vi "Robot Move Board.vi"(9 "Z":dbl, 10 "Value":T1, 11 "Laser Point":cluster{"X":dbl, "Y":dbl, "Angle":dbl}) -> (0 "error out":errorcluster)   [LabVIEW 2019, in "MPC_Laser Marked.lvclass"]
uses:
  MPC_Laser Marked.lvclass
  Function/Main UI/Ctrl/XY Table Action.ctl
  LLB/Commonly VI/FilterPointNameToFloat.vi
  Function/Axis/Axis_Class/SubVI/Axis Motion/Axis_Go Point.vi
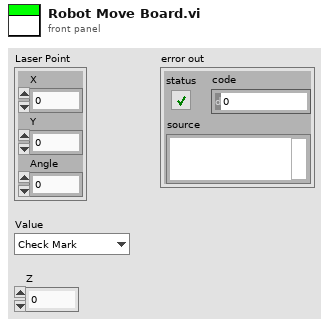
[diagram p1: front panel]
types:
  T1 = typedef "XY Table Action.ctl" = enum16{"Check Mark", "Check Z", "Laser", "Request Action"}
  T2 = enum16{"Initial", "Load", "Save", "Read", "WriteSpeed", "WritePoint"}
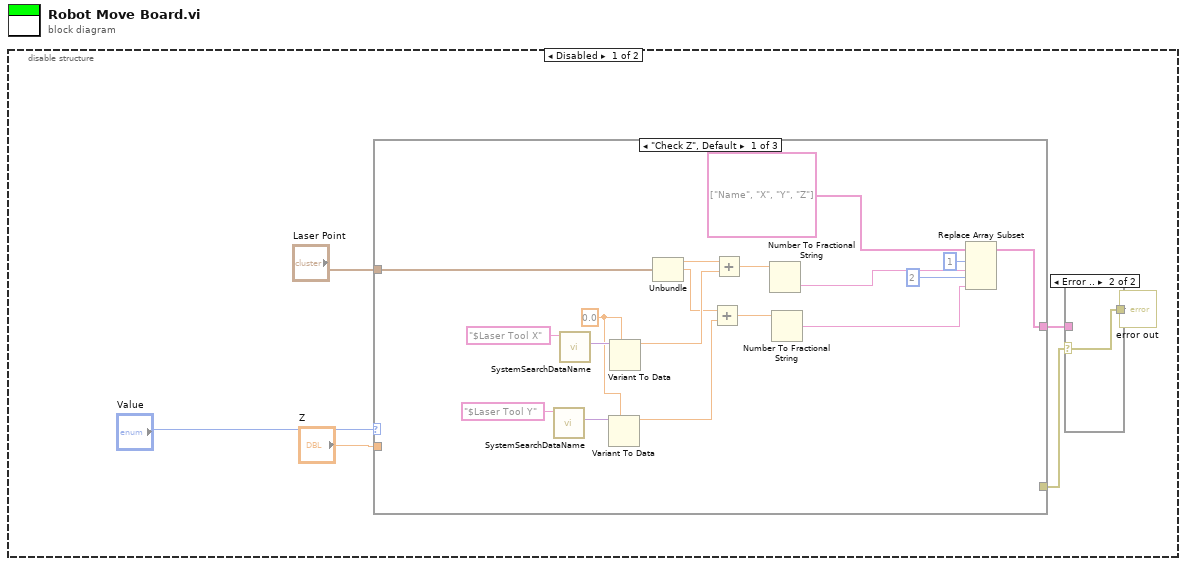
[diagram p0: block diagram]
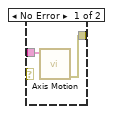
[diagram p2: hidden frame]
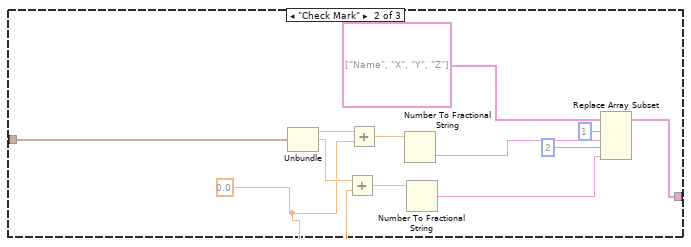
[diagram p3: hidden frame]
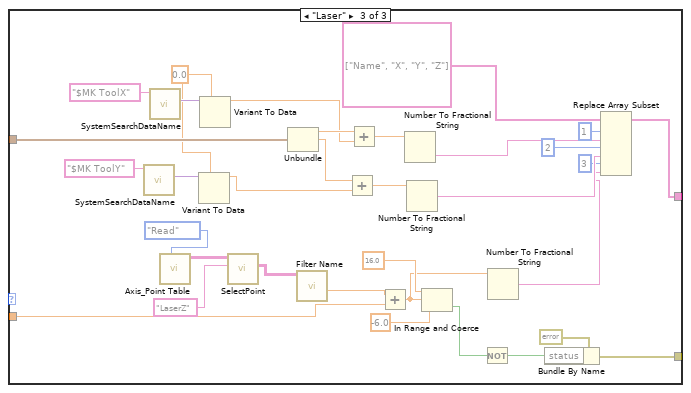
[diagram p4: hidden frame]
diagram:
  n1 = disable-structure shown="Disabled" {
    frame Disabled {
      n2 = case shown="\"Check Z\", Default" "Value" {
        tunnel: [w17 w36 w69] -> w1
        tunnel: "Laser Point" -> [w10 w29 w62]
        tunnel: "Z" -> [_ _ w56]
        tunnel: [_ _ w52] -> w6
        frame "Check Z", Default {
          w23 = 0.0
          n3 = call "SystemSearchDataName.vi"("element"="$Laser Tool Y") -> ("variant"=w24:variant)  [unwired: 8 in, 2 out]
          n4 = call "SystemSearchDataName.vi"("element"="$Laser Tool X") -> ("variant"=w25:variant)  [unwired: 8 in, 2 out]
          n5 = Variant To Data(type=w23, Variant=w24) -> (data=w19:dbl)  [unwired: 1 in, 1 out]
          n6 = Variant To Data(type=w23, Variant=w25) -> (data=w21:dbl)  [unwired: 1 in, 1 out]
          n7 = Unbundle(w10) -> ("X"=w22:dbl, "Y"=w20:dbl)  [unwired: 1 out]
          n8 = Add(x=w20, y=w19) -> (x+y=w15:dbl)
          n9 = Add(x=w22, y=w21) -> (x+y=w16:dbl)
          n10 = Number To Fractional String(number=w16) -> (F-format string=w12:string)  [unwired: 3 in]
          n11 = Number To Fractional String(number=w15) -> (F-format string=w11:string)  [unwired: 3 in]
          n12 = Replace Array Subset(array=string[] ["Name", "X", "Y", "Z"] ("RobotPointsOut"), new element #1=w12, index #1=1 ("index"), new element #2=w11, index #2=2 ("index")) -> (w17:string[])
        }
        frame "Check Mark" {
          w28 = 0.0
          n13 = Unbundle(w29) -> ("X"=w39:dbl, "Y"=w38:dbl)  [unwired: 1 out]
          n14 = Add(x=w38, y=w28) -> (x+y=w34:dbl)
          n15 = Add(x=w39, y=w28) -> (x+y=w35:dbl)
          n16 = Number To Fractional String(number=w35) -> (F-format string=w31:string)  [unwired: 3 in]
          n17 = Number To Fractional String(number=w34) -> (F-format string=w30:string)  [unwired: 3 in]
          n18 = Replace Array Subset(array=string[] ["Name", "X", "Y", "Z"] ("RobotPointsOut"), new element #1=w31, index #1=1 ("index"), new element #2=w30, index #2=2 ("index")) -> (w36:string[])
        }
        frame "Laser" {
          w47 = 0.0
          n19 = call "SystemSearchDataName.vi"("element"="$MK ToolY") -> ("variant"=w48:variant)  [unwired: 8 in, 2 out]
          n20 = call "SystemSearchDataName.vi"("element"="$MK ToolX") -> ("variant"=w49:variant)  [unwired: 8 in, 2 out]
          n21 = call "Axis_Point Table.vi"("Enum"=T2."Read") -> ("RobotPoint"=w61:string[][])  [unwired: 8 in, 2 out]
          n22 = Variant To Data(type=w47, Variant=w48) -> (data=w43:dbl)  [unwired: 1 in, 1 out]
          n23 = Variant To Data(type=w47, Variant=w49) -> (data=w44:dbl)  [unwired: 1 in, 1 out]
          n24 = call "SelectPoint.vi"("PointName"="LaserZ", "RobotPointsTableIn"=w61) -> ("RobotPointsOut"=w58:string[][])  [unwired: 7 in, 2 out]
          n25 = Unbundle(w62) -> ("X"=w72:dbl, "Y"=w71:dbl)  [unwired: 1 out]
          n26 = call-poly "Filter Name.vi"("RobotPoints in"=w58) -> ("Z"=w57:dbl)  [unwired: 4 in, 6 out]
          n27 = Add(x=w71, y=w43) -> (x+y=w67:dbl)
          n28 = Add(x=w72, y=w44) -> (x+y=w68:dbl)
          n29 = Add(x=w57, y=w56) -> (x+y=w41:dbl)
          n30 = Number To Fractional String(number=w68) -> (F-format string=w64:string)  [unwired: 3 in]
          n31 = Number To Fractional String(number=w67) -> (F-format string=w63:string)  [unwired: 3 in]
          n32 = In Range and Coerce(upper limit=16.0 ("y"), x=w41, lower limit=-6.0 ("y")) -> (In Range?=w51:bool)  [unwired: 1 out]
          n33 = Not(x=w51) -> (.not. x?=w50:bool)
          n34 = Number To Fractional String(number=w41) -> (F-format string=w40:string)  [unwired: 3 in]
          n35 = Bundle By Name(cluster=errorcluster {"status"=FALSE, "code"=15010, "source"=""} ("error constant"), "status"=w50) -> (w52:errorcluster)
          n36 = Replace Array Subset(array=string[] ["Name", "X", "Y", "Z"] ("RobotPointsOut"), new element #1=w64, index #1=1 ("index"), new element #2=w63, index #2=2 ("index"), new element #3=w40, index #3=3 ("index")) -> (w69:string[])
        }
      }
      n37 = case shown="Error .." w6 {
        selector: w6 -> [_ w9]
        tunnel: w1 -> [w8 _]
        tunnel: [w7 w9] -> w2
        frame No Error {
          n38 = call-poly "Axis Motion.vi"("RobotPoints in"=w8) -> ("error out"=w7:errorcluster)  [unwired: 10 in]
        }
        frame Error {
        }
      }
      "error out" <- w2
    }
    frame Enabled {
    }
  }
